vi "Array Delta [I32].vi"(2 "Array in":i32[](array[numeric])) -> (7 "Array Delta out":i32[](array[numeric]))   [LabVIEW 2019]
doc: "Computes X[i+1] - X[i] for i = 0 to N-2, where N = size(X)"
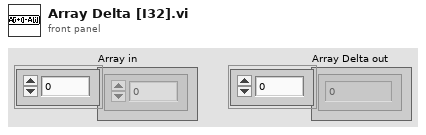
[diagram p1: front panel]
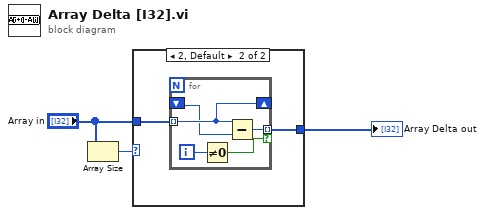
[diagram p0: block diagram]
diagram:
  n1 = Array Size(array="Array in") -> (size(s)=w1:i32)
  n2 = case shown="2, Default" w1 {
    tunnel: [_ w5] -> w3
    tunnel: "Array in" -> [_ w4]
    frame 0, 1 {
    }
    frame 2, Default {
      n3 = for {
        tunnel: w4 -> [w9] mode=indexing
        shift-right: [w9] -> _
        shift-left: _ -> [w8]
        tunnel: [w7] -> w5 mode=indexing if=w6
        i -> [w10]
        n4 = Not Equal To 0?(x=w10) -> (x != 0?=w6:bool)
        n5 = Subtract(x=w9, y=w8) -> (x-y=w7:i32)
      }
    }
  }
  "Array Delta out" <- w3
